vi "outputTOmT.vi"(5 "Input":string, 11 "error in (no error)":errorcluster) -> (6 "Numeric":dbl, 15 "error out":errorcluster)   [LabVIEW 2014, in "FH 55.lvlib"]
uses:
  FH 55.lvlib
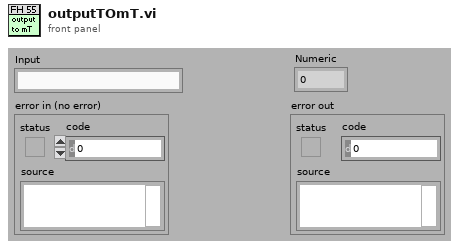
[diagram p1: front panel]
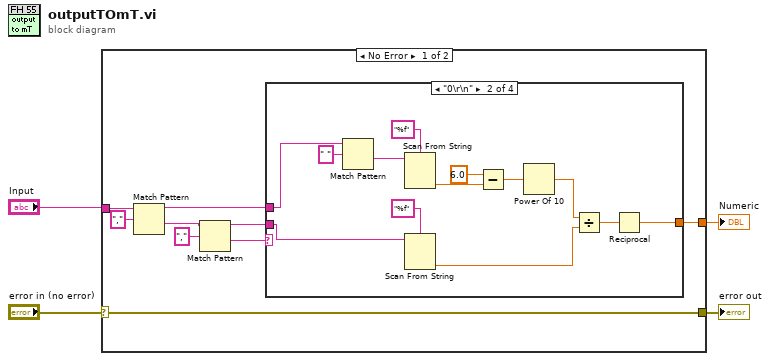
[diagram p0: block diagram]
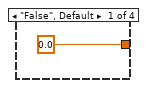
[diagram p2: hidden frame]
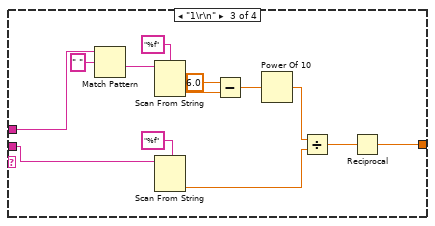
[diagram p3: hidden frame]
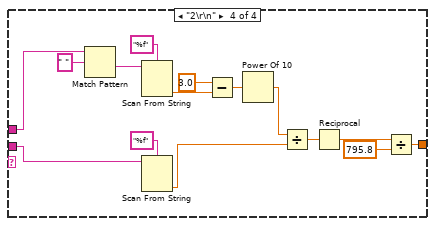
[diagram p4: hidden frame]
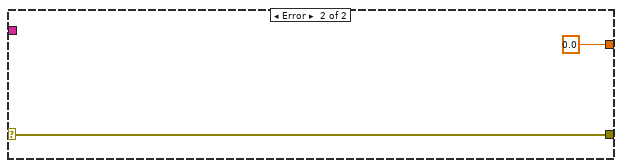
[diagram p5: hidden frame]
diagram:
  n1 = case shown="No Error" "error in (no error)" {
    selector: "error in (no error)" -> [w5 w57]
    tunnel: [w12 0.0] -> w4
    tunnel: [w5 w57] -> w2
    tunnel: "Input" -> [w11 _]
    frame No Error {
      n2 = Match Pattern(string=w11, regular expression=",") -> (before substring=w6:string, after substring=w10:string)  [unwired: 1 in, 2 out]
      n3 = Match Pattern(string=w10, regular expression=",") -> (before substring=w8:string, after substring=w7:string)  [unwired: 1 in, 2 out]
      n4 = case shown="\"0\\r\\n\"" w7 {
        tunnel: [0.0 w16 w29 w49] -> w12
        tunnel: w8 -> [_ w15 w28 w41]
        tunnel: w6 -> [_ w20 w33 w46]
        frame "False", Default {
        }
        frame "0\r\n" {
          n5 = Match Pattern(string=w20, regular expression=" ") -> (after substring=w21:string)  [unwired: 1 in, 3 out]
          n6 = Scan From String(format string="%f", input string=w21) -> (output 1=w24:dbl)  [unwired: 3 in, 3 out]
          n7 = Scan From String(format string="%f", input string=w15) -> (output 1=w18:dbl)  [unwired: 3 in, 3 out]
          n8 = Subtract(x=6.0, y=w24) -> (x-y=w23:dbl)
          n9 = Power Of 10(x=w23) -> (10^x=w19:dbl)
          n10 = Divide(x=w19, y=w18) -> (x/y=w17:dbl)
          n11 = Reciprocal(x=w17) -> (1/x=w16:dbl)
        }
        frame "1\r\n" {
          n12 = Match Pattern(string=w33, regular expression=" ") -> (after substring=w34:string)  [unwired: 1 in, 3 out]
          n13 = Scan From String(format string="%f", input string=w34) -> (output 1=w37:dbl)  [unwired: 3 in, 3 out]
          n14 = Scan From String(format string="%f", input string=w28) -> (output 1=w32:dbl)  [unwired: 3 in, 3 out]
          n15 = Subtract(x=6.0, y=w37) -> (x-y=w36:dbl)
          n16 = Power Of 10(x=w36) -> (10^x=w31:dbl)
          n17 = Divide(x=w31, y=w32) -> (x/y=w30:dbl)
          n18 = Reciprocal(x=w30) -> (1/x=w29:dbl)
        }
        frame "2\r\n" {
          n19 = Match Pattern(string=w46, regular expression=" ") -> (after substring=w47:string)  [unwired: 1 in, 3 out]
          n20 = Scan From String(format string="%f", input string=w47) -> (output 1=w52:dbl)  [unwired: 3 in, 3 out]
          n21 = Scan From String(format string="%f", input string=w41) -> (output 1=w44:dbl)  [unwired: 3 in, 3 out]
          n22 = Subtract(x=3.0, y=w52) -> (x-y=w51:dbl)
          n23 = Power Of 10(x=w51) -> (10^x=w45:dbl)
          n24 = Divide(x=w45, y=w44) -> (x/y=w43:dbl)
          n25 = Reciprocal(x=w43) -> (1/x=w42:dbl)
          n26 = Divide(x=w42, y=795.8) -> (x/y=w49:dbl)
        }
      }
    }
    frame Error {
    }
  }
  "Numeric" <- w4
  "error out" <- w2
